vi "_DSF file transfers to data.vi"(8 "error in (no error)":errorcluster, 10 "group":T5, 11 "configuration file cluster in":T1) -> (0 "error out":errorcluster, 2 "transfers":T9[](array[typedef]), 3 "configuration file cluster out":T1)   [LabVIEW 2017, in "DSF Configuration API v1.0.0.lvlib"]
uses:
  DSF Configuration API v1.0.0.lvlib
  Controls/dsf configuration file/1.0.0/dsf group.ctl
  Controls/dsf configuration file/1.0.0/dsf timing.ctl
  Controls/dsf configuration file/1.0.0/dsf configuration.ctl
  Controls/dsf configuration file/1.0.0/version.ctl
  Controls/dsf configuration file/1.0.0/dsf plugin.ctl
  Controls/dsf configuration file/1.0.0/dsf transfer.ctl
  Controls/dsf configuration file/1.0.0/dsf channel.ctl
  Controls/dsf configuration file/1.0.0/dsf settings.ctl
  Controls/dsf configuration data/1.0.0/dsf transfer.ctl
  Controls/dsf configuration data/1.0.0/dsf channel.ctl
  Controls/dsf configuration data/1.0.0/dsf settings.ctl
  get item value by id/get transfer value by id.vi
  get item value by id/get setting value by id.vi
  Controls/dsf configuration data/1.0.0/dsf configuration data v1.0.0.lvlib
  Controls/dsf configuration file/1.0.0/dsf configuration file v1.0.0.lvlib
panel:
  # "dsf\nfile"
  # "dsf\nfile"
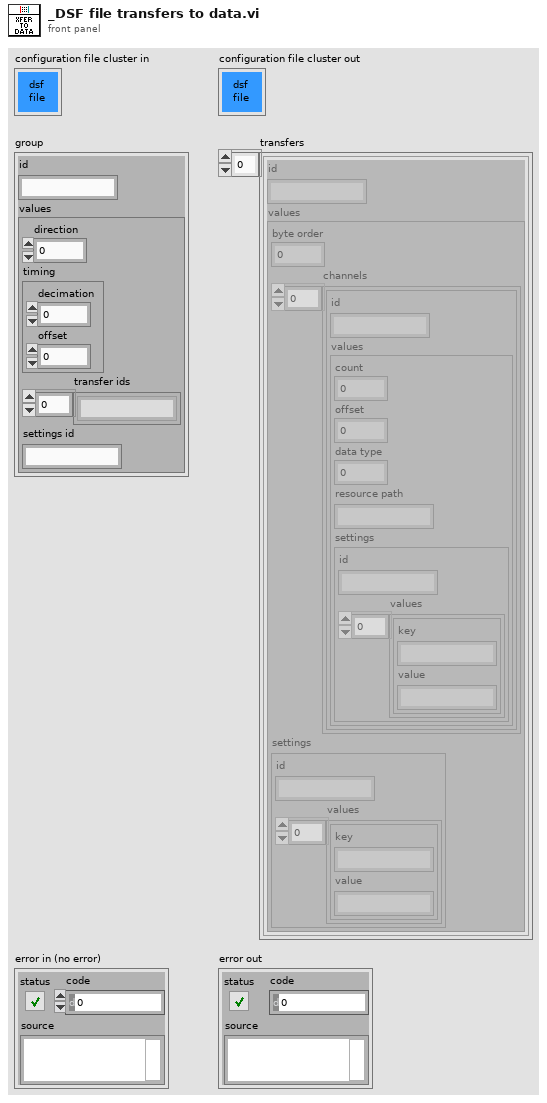
[diagram p1: front panel]
types:
  T1 = typedef "dsf configuration file v1.0.0.lvlib/dsf configuration.ctl" = cluster{"dsf":T2, "configuration":T2, "plugins":T3[], "groups":T5[], "transfers":T6[], "channels":T7[], "settings":T8[]}
  T2 = typedef "dsf configuration file v1.0.0.lvlib/version.ctl" = cluster{"major":u32, "minor":u32, "fix":u32, "build":string}
  T3 = typedef "dsf configuration file v1.0.0.lvlib/dsf plugin.ctl" = cluster{"id":string, "values":cluster{"type":string, "timing":T4, "group ids":string[], "settings id":string}}
  T4 = typedef "dsf configuration file v1.0.0.lvlib/dsf timing.ctl" = cluster{"decimation":i32, "offset":i32}
  T5 = typedef "dsf configuration file v1.0.0.lvlib/dsf group.ctl" = cluster{"id":string, "values":cluster{"direction":i32, "timing":T4, "transfer ids":string[], "settings id":string}}
  T6 = typedef "dsf configuration file v1.0.0.lvlib/dsf transfer.ctl" = cluster{"id":string, "values":cluster{"byte order":i32, "channel ids":string[], "settings id":string}}
  T7 = typedef "dsf configuration file v1.0.0.lvlib/dsf channel.ctl" = cluster{"id":string, "values":cluster{"count":i32, "offset":i32, "data type":i32, "resource path":string, "settings id":string}}
  T8 = typedef "dsf configuration file v1.0.0.lvlib/dsf settings.ctl" = cluster{"id":string, "values":cluster{"key":string, "value":string}[]}
  T9 = typedef "dsf configuration data v1.0.0.lvlib/dsf transfer.ctl" = cluster{"id":string, "values":cluster{"byte order":i32, "channels":T10[], "settings":T11}}
  T10 = typedef "dsf configuration data v1.0.0.lvlib/dsf channel.ctl" = cluster{"id":string, "values":cluster{"count":i32, "offset":i32, "data type":i32, "resource path":string, "settings":T11}}
  T11 = typedef "dsf configuration data v1.0.0.lvlib/dsf settings.ctl" = cluster{"id":string, "values":cluster{"key":string, "value":string}[]}
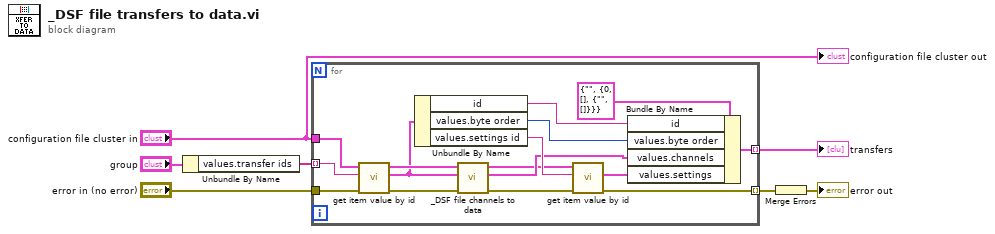
[diagram p0: block diagram]
diagram:
  n1 = Unbundle By Name("group") -> ("values.transfer ids"=w6:string[])
  n2 = for {
    tunnel: "configuration file cluster in" -> [w23]
    tunnel: w6 -> [w22] mode=indexing
    tunnel: [w19] -> w1 mode=indexing
    tunnel: "error in (no error)" -> [w14]
    tunnel: [w11] -> w4 mode=indexing
    n3 = call-poly "get item value by id.vi"("error in (no error)"=w14, "id"=w22, "configuration file cluster in"=w23) -> ("error out"=w13:errorcluster, "transfer"=w10:T6, "configuration file cluster out"=w17:T1)  [unwired: 5 in, 1 out]
    n4 = Unbundle By Name(w10) -> ("id"=w20:string, "values.byte order"=w18:i32, "values.settings id"=w15:string)
    n5 = call "_DSF file channels to data.vi"("error in (no error)"=w13, "transfer"=w10, "configuration file cluster in"=w17) -> ("error out"=w12:errorcluster, "channels"=w9:T10[], "configuration file cluster out"=w8:T1)  [unwired: 6 in]
    n6 = call-poly "get item value by id.vi"("error in (no error)"=w12, "id"=w15, "configuration file cluster in"=w8) -> ("error out"=w11:errorcluster, "settings"=w16:T8)  [unwired: 5 in, 2 out]
    n7 = Bundle By Name(cluster=T9 {"id"="", "values"={"byte order"=0, "channels"=[], "settings"={"id"="", "values"=[]}}} ("transfer"), "id"=w20, "values.byte order"=w18, "values.channels"=w9, "values.settings"=w16) -> (w19:T9)
  }
  "transfers" <- w1
  n8 = Merge Errors(w4) -> (→"error out":errorcluster)
  "configuration file cluster out" <- "configuration file cluster in"
